vi "ChipKit Tone.vi"() -> ()   [LabVIEW 2011, in "LabVIEW Interface for ChipKit.lvlib"]
doc: "An example that uses the Chipkit's digital output pins to generate a tone that can be played on a speaker or piezo buzzer."
uses:
  vi.lib/LabVIEW Interface for ChipKit/LabVIEW Interface for ChipKit.lvlib
  vi.lib/LabVIEW Interface for ChipKit/Private/Type Defs/Board Type.ctl
  vi.lib/LabVIEW Interface for ChipKit/Private/Type Defs/Connection Type.ctl
  vi.lib/LabVIEW Interface for ChipKit/Private/Type Defs/Chipkit Resource.ctl
panel:
  in  "Buzzer Pin":u8=4
  in  "Frequency (0 Hz)":u16(knob)=440 step=100 scale=0.0..20000.0
  in  "ChipKit Configuration":T1={"COM Port"="COM3", "Board Type"=enum."ChipKit uC32", "Connection Type"=enum."USB / Serial", "Baud Rate (115200)"=115200, "Bytes Per Packet (15)"=15, "DI Port Num Pins"=0, "DO Port Num Pins"=0}
  in  "Stop Button":bool
  # "chipKIT Settings"
  # "Speaker Settings"
  # "Piezo Buzzer Tone Example\n\nThis example demonstrates how generate an audio tone using a piezo buzzer.\n\nInstructions\n1. Select the COM Port associated with the ChipKit.\n2. Select the Board Type.\n3. Select the Buzzer Pin connected to the piezo buzzer.\n4. Click the Run Arrow.\n5. Adjust the Frequency control to change the pitch of the generated audio tone."
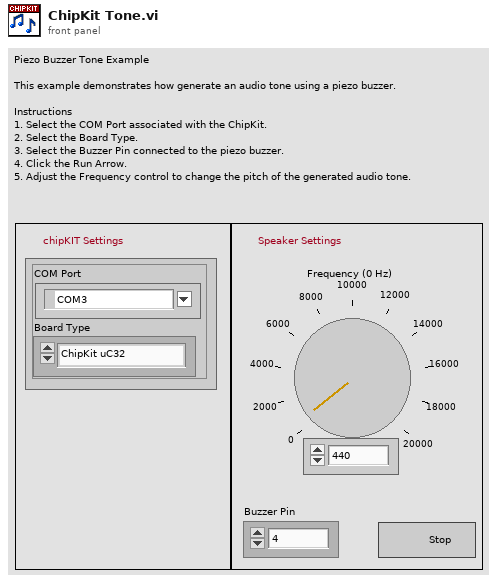
[diagram p1: front panel]
types:
  T1 = typedef "LabVIEW Interface for ChipKit.lvlib/Chipkit Resource.ctl" = cluster{"COM Port":refnum<visa-resource-name>, "Board Type":T2, "Connection Type":T3, "Baud Rate (115200)":u32, "Bytes Per Packet (15)":u32, "DI Port Num Pins":i32, "DO Port Num Pins":i32}
  T2 = typedef "LabVIEW Interface for ChipKit.lvlib/Board Type.ctl" = enum16{"ChipKit uC32", "ChipKit Uno32", "ChipKit Max32"}
  T3 = typedef "LabVIEW Interface for ChipKit.lvlib/Connection Type.ctl" = enum8{"USB / Serial", "XBEE", "BlueSmirf (Bluetooth)"}
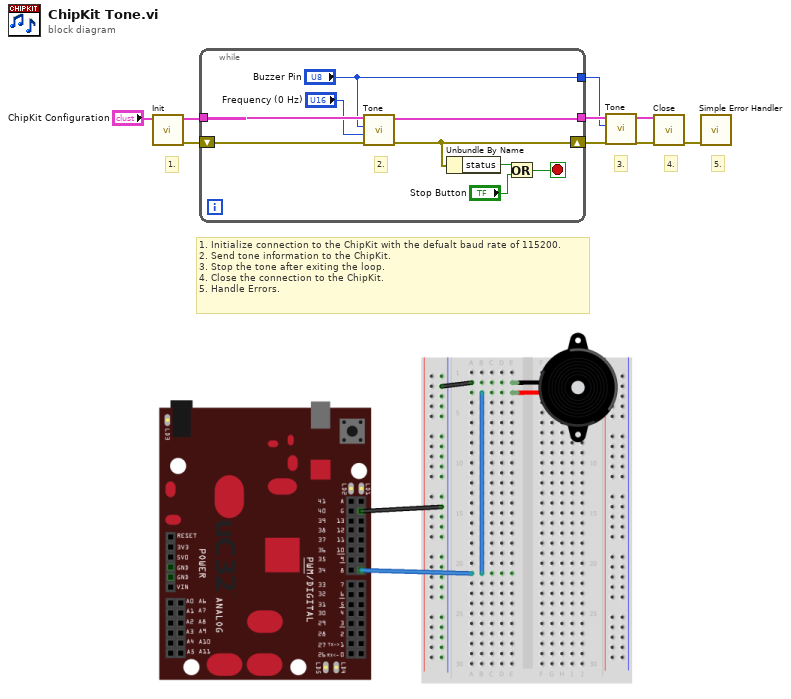
[diagram p0: block diagram]
diagram:
  # "5."
  # "1. Initialize connection to the ChipKit with the defualt baud rate of 115200.\n2. Send tone information to the ChipKit.\n3. Stop the tone after exiting the loop.\n4. Close the connection to the ChipKit.\n5. Handle Errors."
  # "4."
  # "3."
  # "1."
  n1 = call "Init.vi"("ChipKit Configuration"="ChipKit Configuration") -> ("Error Out"=w8:errorcluster, "ChipKit Configuration"=w9:T1)  [unwired: 9 in]
  n2 = while {
    tunnel: w9 -> [w16]
    shift-right: [w13] -> w5
    shift-left: w8 -> [w15]
    tunnel: [w14] -> w4
    tunnel: ["Buzzer Pin"] -> w1
    stop <- w18 stop-if-true
    # "2."
    n3 = call "Tone.vi"("Error In"=w15, "Frequency (0 Hz)"="Frequency (0 Hz)", "Buzzer Pin"="Buzzer Pin", "ChipKit Resource"=w16) -> ("Error Out"=w13:errorcluster, "ChipKit Resource"=w14:T1)  [unwired: 6 in]
    n4 = Unbundle By Name(w13) -> ("status"=w17:bool)
    n5 = Or(x=w17, y="Stop Button") -> (x .or. y?=w18:bool)
  }
  n6 = call "Tone.vi"("Error In"=w5, "Buzzer Pin"=w1, "ChipKit Resource"=w4) -> ("Error Out"=w2:errorcluster, "ChipKit Resource"=w3:T1)  [unwired: 7 in]
  n7 = call "Close.vi"("Error In"=w2, "ChipKit Configuration"=w3) -> ("Error Out"=w7:errorcluster)  [unwired: 9 in]
  n8 = call <vilib>:"Simple Error Handler.vi"("error in (no error)"=w7) -> ()  [unwired: 4 in, 5 out]
